vi "Read Size Height.vi"(8 "error in (no error)":errorcluster, 11 "IOName.lvclass in":refnum<class "IOName.lvclass">) -> (0 "error out":errorcluster, 2 "Height":u32, 3 "IOName.lvclass out":refnum<class "IOName.lvclass">)   [LabVIEW 2015, in "IOName.lvclass"]
uses:
  IOName.lvclass
  IOName.lvclass/IOName.ctl
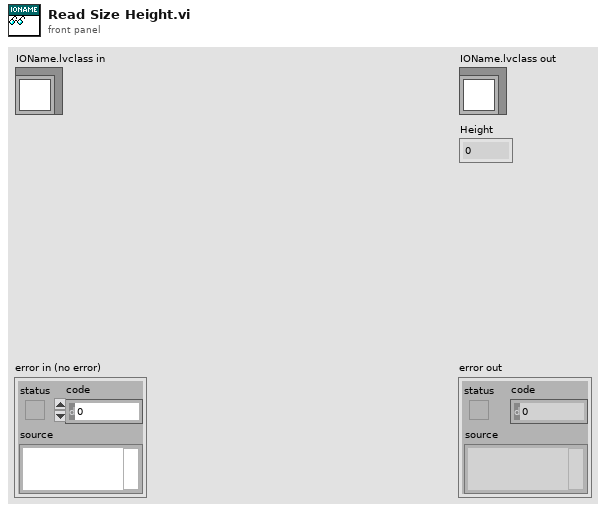
[diagram p1: front panel]
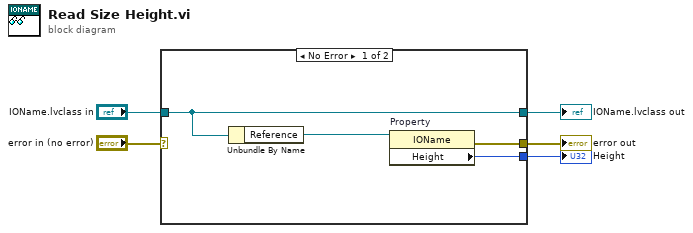
[diagram p0: block diagram]
diagram:
  n1 = case shown="No Error" "error in (no error)" {
    selector: "error in (no error)" -> [_ w11]
    tunnel: [w8 w11] -> w4
    tunnel: [w7 w10] -> w2
    tunnel: "IOName.lvclass in" -> [w7 w10]
    tunnel: [w9 _] -> w1
    frame No Error {
      n2 = Unbundle By Name(w7) -> ("Reference"=w6:refnum<vi>)
      n3 = property on="Property" class="IOName"(reference=w6) -> (error out=w8:errorcluster, "Height"=w9:u32)  [unwired: 1 in, 1 out]
    }
    frame Error {
    }
  }
  "error out" <- w4
  "IOName.lvclass out" <- w2
  "Height" <- w1
